vi "Expand FIFO Type Def Init.vi"(8 "error in (no error)":errorcluster, 9 "Current Bus Number":i32, 10 "Path to All Nodes Resources":string, 11 "Destination Path":path) -> (0 "error out":errorcluster, 3 "Cluster out":refnum<vi>, 5 "Control Refnum":refnum<vi>)   [LabVIEW 2014, in "Initialization and IO Node Scripting.lvlib"]
uses:
  Initialization and IO Node Scripting.lvlib
  <vilib>/Utility/traverseref.llb/TRef TravTarget.ctl
  <vilib>/Utility/traverseref.llb/VI Scripting - Traverse.lvlib
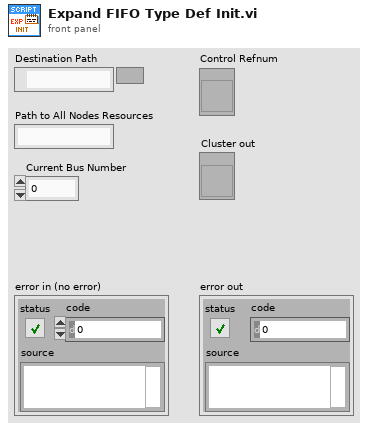
[diagram p1: front panel]
types:
  T1 = typedef "TRef TravTarget.ctl" = enum16{"FP", "BD", "Other"}
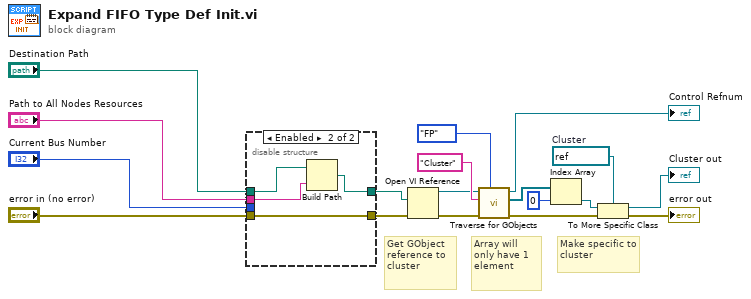
[diagram p0: block diagram]
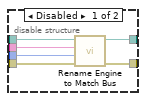
[diagram p2: hidden frame]
diagram:
  w8 = refnum<vi> refnum  # Cluster
  # "Array will only have 1 element"
  # "Make specific to cluster"
  # "Get GObject reference to cluster"
  n1 = disable-structure shown="Enabled" {
    disable-tunnel: "error in (no error)" -> [w24 w26]
    disable-tunnel: [w23 w26] -> w5
    disable-tunnel: "Destination Path" -> [w22 w28]
    disable-tunnel: "Path to All Nodes Resources" -> [w21 w27]
    disable-tunnel: [w20 w25] -> w2
    disable-tunnel: "Current Bus Number" -> [w19 _]
    frame Disabled {
      n2 = call "Rename Engine to Match Bus.vi"("error in (no error)"=w24, "Current Bus Number"=w19, "Path to File"=w21, "Current Bus Path"=w22) -> ("error out"=w23:errorcluster, "New File Path"=w20:path)  [unwired: 6 in]
    }
    frame Enabled {
      n3 = Build Path(base path=w28, name or relative path=w27) -> (appended path=w25:path)
    }
  }
  n4 = Open VI Reference(vi path=w2, error in (no error)=w5) -> (vi reference=w12:refnum<vi>, error out=w15:errorcluster)  [unwired: 4 in]
  n5 = call <vilib>:"Traverse for GObjects.vi"("Traverse Target"=TRef_TravTarget."FP", "error in (no error)"=w15, "Class Name"="Cluster", "VI Refnum"=w12) -> ("error out"=w16:errorcluster, "References"=w11:refnum<vi>[], "dup VI Refnum"=→"Control Refnum":refnum<vi>)  [unwired: 4 in, 1 out]
  n6 = Index Array(array=w11, index=0) -> (element=w9:refnum<vi>)
  n7 = To More Specific Class(target class=w8, reference=w9, error in=w16) -> (specific class reference=→"Cluster out":refnum<vi>, error out=→"error out":errorcluster)
